vi "oa_Create Indice.vi"(0 "X axis selection":u16(ring)=2 items=["Time", "Revolution", "RPM"], 1 "reset?(F)":bool, 5 "step found?(F)":bool, 7 "steps input":cluster{"start":dbl, "end":dbl, "step":dbl} {"step" format="%.2f"; "end" format="%.2f"; "start" format="%.2f"}, 9 "speed profile":cluster{"time [s]":dbl[], "speed [RPM]":dbl[]} {"speed [RPM]" format="%.2f"; "time [s]" format="%.2f"}, 11 "error in (no error)":errorcluster, 12 "pulse/revolution (1)":i32=1) -> (3 "last rev":dbl, 4 "rev indice":dbl[](array[numeric]), 6 "time indice":dbl[](array[numeric]), 8 "RPM indice":dbl[](array[numeric]), 10 "scale":cluster{"offset":dbl, "multiplier":dbl}, 14 "reach end?":bool, 15 "error out":errorcluster)   [LabVIEW 2017]
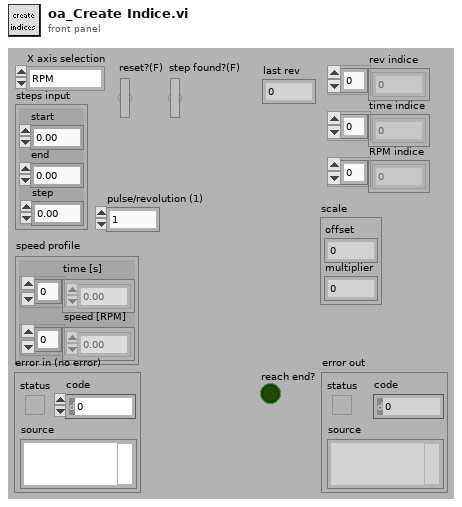
[diagram p1: front panel]
types:
  T1 = cluster{"start":dbl, "# of steps":i32, "step":dbl}
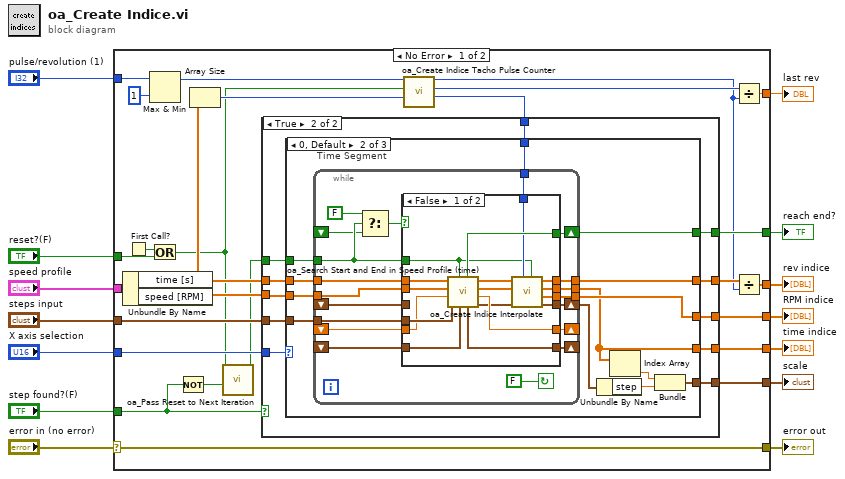
[diagram p0: block diagram]
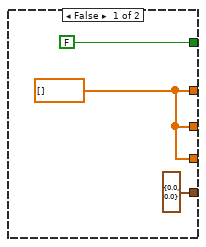
[diagram p2: hidden frame]
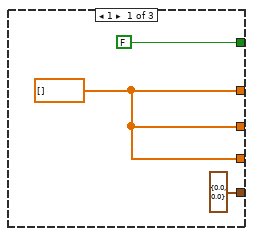
[diagram p3: hidden frame]
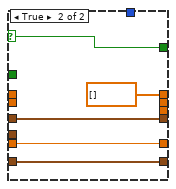
[diagram p4: hidden frame]
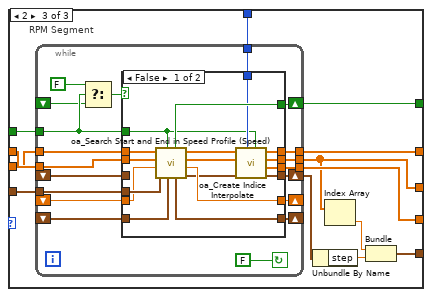
[diagram p5: hidden frame]
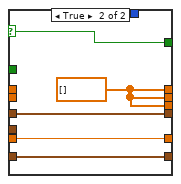
[diagram p6: hidden frame]
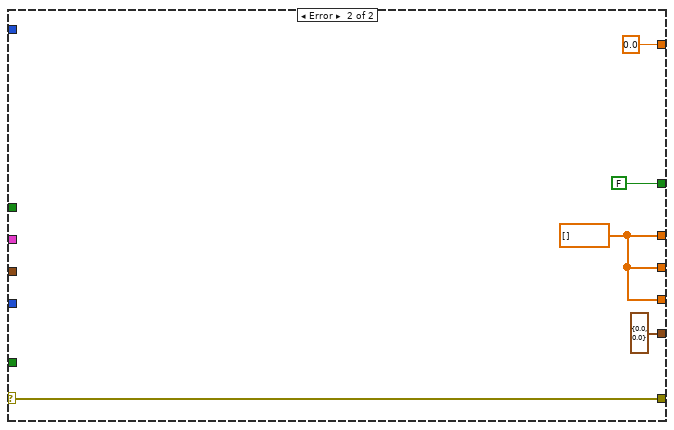
[diagram p7: hidden frame]
diagram:
  n1 = case shown="No Error" "error in (no error)" {
    selector: "error in (no error)" -> [w39 w169]
    tunnel: [w39 w169] -> w12
    tunnel: "X axis selection" -> [w38 _]
    tunnel: "steps input" -> [w37 _]
    tunnel: "speed profile" -> [w33 _]
    tunnel: "reset?(F)" -> [w29 _]
    tunnel: [w36 FALSE] -> w8
    tunnel: [w35 w166] -> w7
    tunnel: [w34 w166] -> w6
    tunnel: [w25 w166] -> w5
    tunnel: [w28 0.0] -> w4
    tunnel: "step found?(F)" -> [w20 _]
    tunnel: "pulse/revolution (1)" -> [w23 _]
    tunnel: [w17 cluster{dbl, "step":dbl} {0.0, "step"=0.0}] -> w1
    frame No Error {
      n2 = Unbundle By Name(w33) -> ("time [s]"=w31:dbl[], "speed [RPM]"=w32:dbl[])
      n3 = First Call?() -> (First Call?: T/F=w30:bool)
      n4 = Max & Min(x=w23, y=1) -> (max(x,y)=w22:i32)  [unwired: 1 out]
      n5 = Or(x=w30, y=w29) -> (x .or. y?=w15:bool)
      n6 = Not(x=w20) -> (.not. x?=w19:bool)
      n7 = Array Size(array=w31) -> (size(s)=w21:i32)
      n8 = call <vilib>:"oa_Pass Reset to Next Iteration.vi"("trigger"=w19, "reset?(F)"=w15) -> ("reset out"=w16:bool)  [unwired: 9 in]
      n9 = call <vilib>:"oa_Create Indice Tacho Pulse Counter.vi"("length"=w21, "reset?"=w15) -> ("tacho pulse passed last round"=w18:i32, "tacho pulse passed"=w27:i32)  [unwired: 8 in]
      n10 = case shown="True" w20 {
        tunnel: w38 -> [_ w53]
        tunnel: w37 -> [_ w45]
        tunnel: [FALSE w52] -> w36
        tunnel: [w41 w51] -> w35
        tunnel: [w41 w50] -> w34
        tunnel: [w41 w49] -> w26
        tunnel: w32 -> [_ w48]
        tunnel: w31 -> [_ w47]
        tunnel: w18 -> [_ w46]
        tunnel: w16 -> [_ w44]
        tunnel: [cluster{dbl, "step":dbl} {0.0, "step"=0.0} w43] -> w17
        frame False {
          w41 = dbl[] []
        }
        frame True {
          n11 = case shown="0, Default" w53 {
            tunnel: w47 -> [_ w69 w121]
            tunnel: w48 -> [_ w68 w120]
            tunnel: w44 -> [_ w67 w122]
            tunnel: [FALSE w64 w119] -> w52
            tunnel: [w55 w62 w112] -> w51
            tunnel: [w55 w59 w117] -> w50
            tunnel: [w55 w63 w118] -> w49
            tunnel: w46 -> [_ w66 w116]
            tunnel: w45 -> [_ w65 w123]
            tunnel: [cluster{dbl, "step":dbl} {0.0, "step"=0.0} w57 w113] -> w43
            frame 1 {
              w55 = dbl[] [] ("revolution indices")
            }
            frame 0, Default {
              # "Time Segment"
              n12 = while {
                tunnel: w69 -> [w86]
                tunnel: w68 -> [w85]
                tunnel: w67 -> [w78]
                tunnel: w66 -> [w87]
                tunnel: w65 -> [w84]
                shift-right: [w83] -> _
                shift-left: _ -> [w82]
                shift-right: [w80] -> _
                shift-left: _ -> [w81]
                shift-right: [w79] -> w64
                shift-left: _ -> [w77]
                tunnel: [w74] -> w63
                tunnel: [w73] -> w59
                tunnel: [w72] -> w62
                shift-right: [w71] -> w61
                shift-left: _ -> [w70]
                stop <- FALSE continue-if-true
                n13 = Select(t=FALSE, s=w78, f=w77) -> (s? t:f=w75:bool)
                n14 = case shown="False" w75 {
                  selector: w75 -> [_ w108]
                  tunnel: w87 -> [w94 _]
                  tunnel: w86 -> [w105 _]
                  tunnel: w85 -> [w104 _]
                  tunnel: w84 -> [w103 _]
                  tunnel: [w102 w110] -> w83
                  tunnel: w82 -> [w101 w110]
                  tunnel: w81 -> [w100 w109]
                  tunnel: [w99 w109] -> w80
                  tunnel: [w98 w108] -> w79
                  tunnel: w78 -> [w90 _]
                  tunnel: [w93 w107] -> w74
                  tunnel: [w92 w107] -> w73
                  tunnel: [w91 w107] -> w72
                  tunnel: [w89 w106] -> w71
                  tunnel: w70 -> [_ w106]
                  frame False {
                    n15 = call <vilib>:"oa_Search Start and End in Speed Profile (time).vi"("last value in"=w100, "reset"=w90, "steps input"=w103, "next value in"=w101, "interpolation array"=w104, "reference array"=w105) -> ("actual steps"=w95:T1, "next value out"=w102:dbl, "interpolation array out"=w96:dbl[], "reference array out"=w97:dbl[], "last value out"=w99:cluster{"reference":dbl, "interpolation":dbl}, "reach end?"=w98:bool)
                    n16 = call <vilib>:"oa_Create Indice Interpolate.vi"("reset?(F)"=w90, "history rev length"=w94, "actual steps"=w95, "interpolation array"=w96, "reference array"=w97) -> ("dup actual steps"=w89:T1, "interpolated values"=w91:dbl[], "reference values"=w92:dbl[], "revolution indices"=w93:dbl[])  [unwired: 3 in]
                  }
                  frame True {
                    w107 = dbl[] [] ("revolution indices")
                  }
                }
              }
              n17 = Unbundle By Name(w61) -> ("step"=w60:dbl)
              n18 = Index Array(array=w59) -> (element=w58:dbl)  [unwired: 1 in]
              n19 = Bundle(w58, "step"=w60) -> (w57:cluster{dbl, "step":dbl})  [unwired: 1 in]
            }
            frame 2 {
              # "RPM Segment"
              n20 = while {
                tunnel: w120 -> [w140]
                tunnel: w121 -> [w139]
                tunnel: w122 -> [w132]
                tunnel: w116 -> [w141]
                tunnel: w123 -> [w138]
                shift-right: [w137] -> _
                shift-left: _ -> [w136]
                shift-right: [w134] -> _
                shift-left: _ -> [w135]
                shift-right: [w133] -> w119
                shift-left: _ -> [w131]
                tunnel: [w128] -> w118
                tunnel: [w127] -> w112
                tunnel: [w126] -> w117
                shift-right: [w125] -> w115
                shift-left: _ -> [w124]
                stop <- FALSE continue-if-true
                n21 = Select(t=FALSE, s=w132, f=w131) -> (s? t:f=w129:bool)
                n22 = case shown="False" w129 {
                  selector: w129 -> [_ w162]
                  tunnel: w141 -> [w148 _]
                  tunnel: w140 -> [w159 _]
                  tunnel: w139 -> [w158 _]
                  tunnel: w138 -> [w157 _]
                  tunnel: [w156 w164] -> w137
                  tunnel: w136 -> [w155 w164]
                  tunnel: w135 -> [w154 w163]
                  tunnel: [w153 w163] -> w134
                  tunnel: [w152 w162] -> w133
                  tunnel: w132 -> [w144 _]
                  tunnel: [w147 w161] -> w128
                  tunnel: [w146 w161] -> w127
                  tunnel: [w145 w161] -> w126
                  tunnel: [w143 w160] -> w125
                  tunnel: w124 -> [_ w160]
                  frame False {
                    n23 = call <vilib>:"oa_Search Start and End in Speed Profile (Speed).vi"("last value in"=w154, "reset"=w144, "steps input"=w157, "next value in"=w155, "interpolation array"=w158, "reference array"=w159) -> ("actual steps"=w149:T1, "next value out"=w156:dbl, "interpolation array out"=w150:dbl[], "reference array out"=w151:dbl[], "last value out"=w153:cluster{"reference":dbl, "interpolation":dbl}, "reach end?"=w152:bool)
                    n24 = call <vilib>:"oa_Create Indice Interpolate.vi"("reset?(F)"=w144, "history rev length"=w148, "actual steps"=w149, "interpolation array"=w150, "reference array"=w151) -> ("dup actual steps"=w143:T1, "interpolated values"=w145:dbl[], "reference values"=w146:dbl[], "revolution indices"=w147:dbl[])  [unwired: 3 in]
                  }
                  frame True {
                    w161 = dbl[] [] ("revolution indices")
                  }
                }
              }
              n25 = Unbundle By Name(w115) -> ("step"=w114:dbl)
              n26 = Index Array(array=w112) -> (element=w111:dbl)  [unwired: 1 in]
              n27 = Bundle(w111, "step"=w114) -> (w113:cluster{dbl, "step":dbl})  [unwired: 1 in]
            }
          }
        }
      }
      n28 = Divide(x=w27, y=w22) -> (x/y=w28:dbl)
      n29 = Divide(x=w26, y=w22) -> (x/y=w25:dbl[])
    }
    frame Error {
      w166 = dbl[] []
    }
  }
  "error out" <- w12
  "reach end?" <- w8
  "RPM indice" <- w7
  "time indice" <- w6
  "rev indice" <- w5
  "last rev" <- w4
  "scale" <- w1
